vi "OpenSF.vi"(0 "Port number":u16) -> (1 "connection ID":refnum<k5>, 2 "Error out":errorcluster)   [LabVIEW 2013]
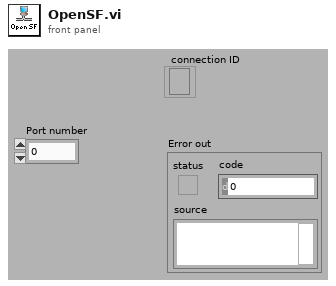
[diagram p1: front panel]
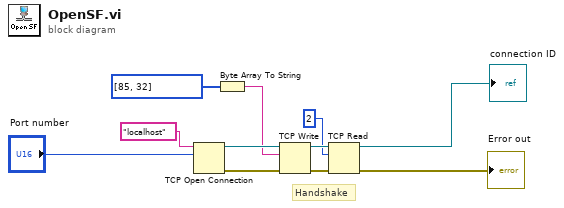
[diagram p0: block diagram]
diagram:
  # "Handshake"
  n1 = TCP Open Connection(address="localhost", remote port or service name="Port number") -> (connection ID=w6:refnum<k5>, error out=w5:errorcluster)  [unwired: 3 in]
  n2 = Byte Array To String(unsigned byte array=u8[] [85, 32]) -> (string=w2:string)
  n3 = TCP Write(connection ID=w6, data in=w2, error in (no error)=w5) -> (connection ID out=w7:refnum<k5>, error out=w8:errorcluster)  [unwired: 1 in, 1 out]
  n4 = TCP Read(connection ID=w7, bytes to read=2, error in (no error)=w8) -> (connection ID out=→"connection ID":refnum<k5>, error out=→"Error out":errorcluster)  [unwired: 2 in, 1 out]
